vi "ELVIS III v1.0 Unreserve Channel List.vi"(7 "Allow multiple opens?":bool, 8 "error in (no error)":errorcluster, 10 "Channel Reservation List":T1, 11 "Owner":string) -> (0 "error out":errorcluster)   [LabVIEW 2021]
uses:
  <vilib>/myRIO/Common/Instrument Driver Framework/ELVIS III v1.0/Resource Manager/typedefs/ELVIS III v1.0 Channel Reservation List.ctl
  <vilib>/myRIO/Common/Instrument Driver Framework/ELVIS III v1.0/Resource Manager/typedefs/ELVIS III v1.0 Channel Reservation Info.ctl
  <vilib>/myRIO/Common/Instrument Driver Framework/ELVIS III v1.0/Resource Manager/typedefs/ELVIS III v1.0 Connector List.ctl
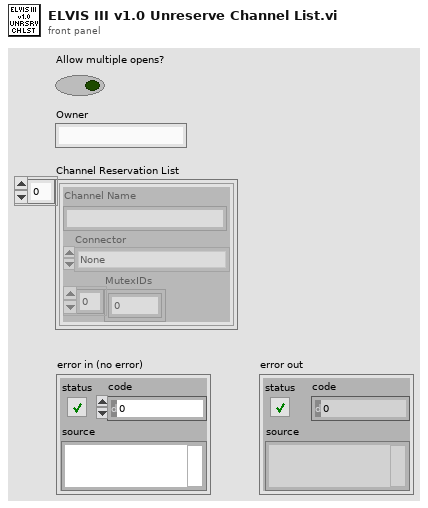
[diagram p1: front panel]
types:
  T1 = typedef "ELVIS III v1.0 Channel Reservation List.ctl" = T2[]
  T2 = typedef "ELVIS III v1.0 Channel Reservation Info.ctl" = cluster{"Channel Name":string, "Connector":T3, "MutexIDs":u32[]}
  T3 = typedef "ELVIS III v1.0 Connector List.ctl" = enum32{"None", "ConnectorA", "ConnectorB"}
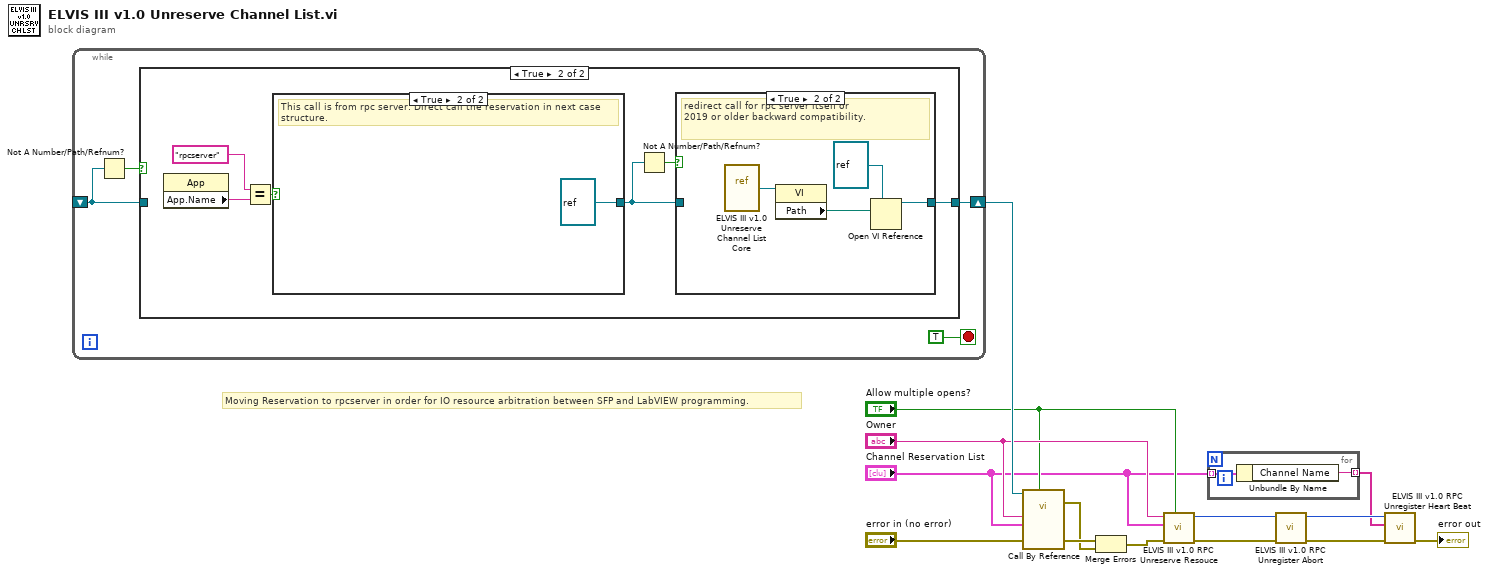
[diagram p0: block diagram]
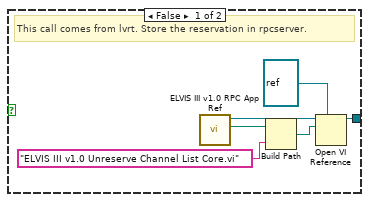
[diagram p4: hidden frame]
diagram:
  # "Moving Reservation to rpcserver in order for IO resource arbitration between SFP and LabVIEW programming."
  n1 = while {
    shift-right: [w17] -> w13
    shift-left: _ -> [w14]
    stop <- TRUE stop-if-true
    n2 = Not A Number/Path/Refnum?(number/path/refnum=w14) -> (NaN/Path/Refnum?=w15:bool)
    n3 = case shown="True" w15 {
      tunnel: [w18 w19] -> w17
      tunnel: w14 -> [w18 _]
      frame False {
      }
      frame True {
        n4 = property class="App"() -> ("App.Name"=w24:string)  [unwired: 2 in, 2 out]
        n5 = Equal?(x="rpcserver" ("Application:Name"), y=w24) -> (x = y?=w23:bool)
        n6 = case shown="True" w23 {
          tunnel: [w34 refnum<vi> refnum ("type specifier VI Refnum (for type only)")] -> w20
          frame False {
            # "This call comes from lvrt. Store the reservation in rpcserver."
            n7 = call <vilib>:"ELVIS III v1.0 RPC App Ref.vi"() -> ("Lib Path"=w33:path, "RPC Reference"=w31:refnum<vi>)  [unwired: 10 in]
            n8 = Build Path(base path=w33, name or relative path="ELVIS III v1.0 Unreserve Channel List Core.vi") -> (appended path=w30:path)
            n9 = Open VI Reference(type specifier VI Refnum (for type only)=refnum<vi> refnum, application reference (local)=w31, vi path=w30) -> (vi reference=w34:refnum<vi>)  [unwired: 3 in, 1 out]
          }
          frame True {
            # "This call is from rpc server. Direct call the reservation in next case structure."
          }
        }
        n10 = Not A Number/Path/Refnum?(number/path/refnum=w20) -> (NaN/Path/Refnum?=w21:bool)
        n11 = case shown="True" w21 {
          tunnel: w20 -> [w25 _]
          tunnel: [w25 w27] -> w19
          frame False {
          }
          frame True {
            # "redirect call for rpc server itself or\n2019 or older backward compatibility."
            n12 = vi-ref <vilib>:"ELVIS III v1.0 Unreserve Channel List Core.vi"() -> (w29:refnum<vi>)
            n13 = property class="VI"(reference=w29) -> ("Path"=w28:path)  [unwired: 1 in, 2 out]
            n14 = Open VI Reference(type specifier VI Refnum (for type only)=refnum<vi> refnum, vi path=w28) -> (vi reference=w27:refnum<vi>)  [unwired: 4 in, 1 out]
          }
        }
      }
    }
  }
  n15 = call-by-ref "?"(reference=w13, "Allow multiple opens?"="Allow multiple opens?", "error in (no error)"="error in (no error)", "Channel Reservation List"="Channel Reservation List", "Owner"="Owner") -> (error out=w1:errorcluster, 0:"error out"=w3:errorcluster)  [unwired: 8 in, 1 out]
  n16 = Merge Errors(w3, w1) -> (w2:errorcluster)
  n17 = call <vilib>:"ELVIS III v1.0 RPC Unreserve Resouce.vi"("Allow multiple opens?"="Allow multiple opens?", "error in (no error)"=w2, "Channel Reservation List"="Channel Reservation List", "Owner"="Owner") -> ("error out"=w9:errorcluster, "Session"=w6:u32)  [unwired: 6 in]
  n18 = for {
    tunnel: "Channel Reservation List" -> [w38] mode=indexing
    tunnel: [w37] -> w4 mode=indexing
    n19 = Unbundle By Name(w38) -> ("Channel Name"=w37:string)
  }
  n20 = call <vilib>:"ELVIS III v1.0 RPC Unregister Abort.vi"("error in (no error)"=w9, "Session"=w6) -> ("error out"=w8:errorcluster)  [unwired: 9 in]
  n21 = call <vilib>:"ELVIS III v1.0 RPC Unregister Heart Beat.vi"("error in (no error)"=w8, "Channel Names"=w4, "Session"=w6) -> ("error out"=→"error out":errorcluster)  [unwired: 8 in]
